vi "APS line all.vi"(0 "Dimension":i32, 1 "Axis_ID_Array":i32, 2 "Option":i32, 3 "PositionArray":dbl, 4 "TransPara":dbl, 5 "Vs":dbl, 6 "Vm":dbl, 7 "error in (no error)":errorcluster caption="错误输入（无错误）", 8 "Ve":dbl, 9 "Acc":dbl, 10 "Dec":dbl, 11 "SFac":dbl, 12 "Wait":cluster{"h_event":u32, "i32_ret":i32}) -> (14 "Wait out":cluster{"h_event":u32, "i32_ret":i32}, 20 "function return":i32, 21 "Axis_ID_Array out":i32, 23 "PositionArray out":dbl, 24 "TransPara out":dbl, 27 "error out":errorcluster caption="错误输出")   [LabVIEW 2011, in "APS168.lvlib"]
doc: "I32 FNTYPE APS_line_all( I32 Dimension, I32 *Axis_ID_Array, I32 Option, F64 *PositionArray, F64 *TransPara, F64 Vs, F64 Vm, F64 Ve, F64 Acc,F64 Dec, F64 SFac, ASYNCALL *Wait);"
uses:
  APS168.lvlib
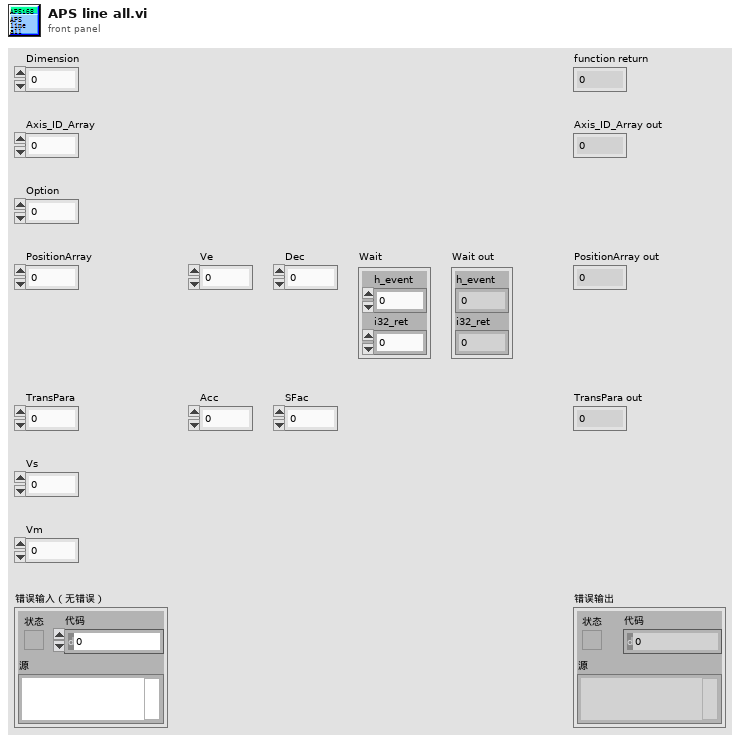
[diagram p1: front panel]
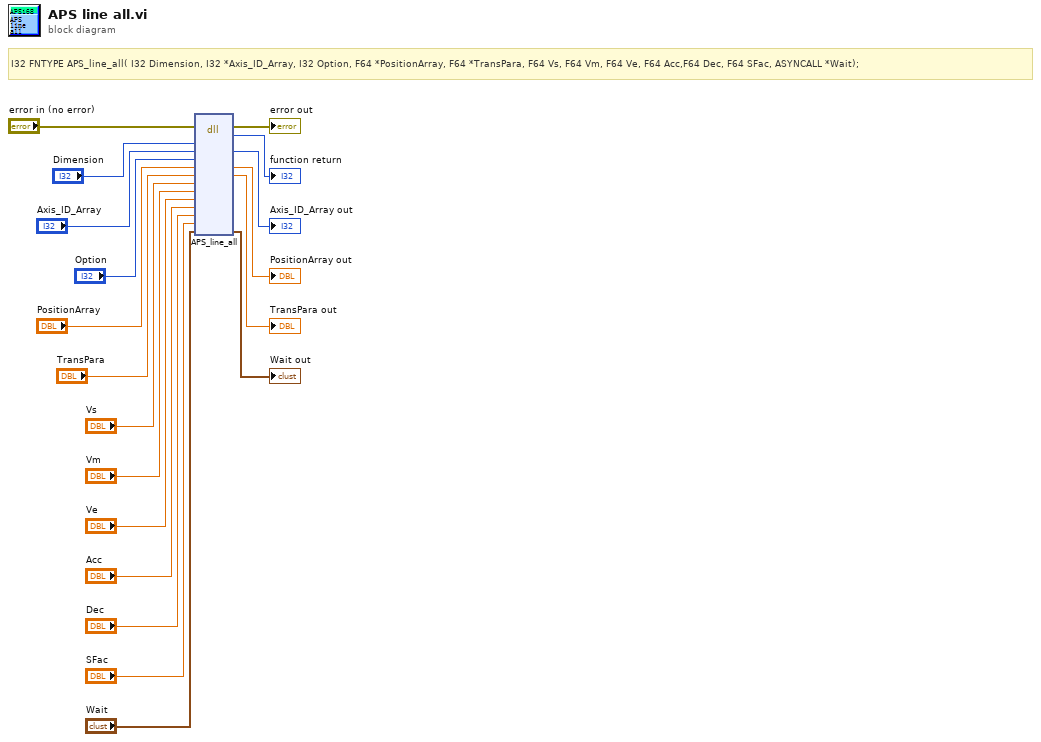
[diagram p0: block diagram]
diagram:
  # "I32 FNTYPE APS_line_all( I32 Dimension, I32 *Axis_ID_Array, I32 Option, F64 *PositionArray, F64 *TransPara, F64 Vs, F64 Vm, F64 Ve, F64 Acc,F64 Dec, F64 SFac, ASYNCALL *Wait);"
  n1 = dll-call lib="PTH1Labs E软件ADLINK 204CAPS_1_7_1_LIB line 连续运动204APS168.*" fn="APS_line_all"(error in="error in (no error)", "Dimension"="Dimension", "Axis_ID_Array"="Axis_ID_Array", "Option"="Option", "PositionArray"="PositionArray", "TransPara"="TransPara", "Vs"="Vs", "Vm"="Vm", "Ve"="Ve", "Acc"="Acc", "Dec"="Dec", "SFac"="SFac", "Wait"="Wait") -> (error out=→"error out":errorcluster, →"function return":i32, "Axis_ID_Array"=→"Axis_ID_Array out":i32, "PositionArray"=→"PositionArray out":dbl, "TransPara"=→"TransPara out":dbl, "Wait"=→"Wait out":cluster{"h_event":u32, "i32_ret":i32})  [unwired: 10 in, 1 out]
